vi "Encoders.vi"(0 "DigitalInputs":bool[](array[boolean])=[FALSE, FALSE, FALSE, FALSE, FALSE, FALSE, FALSE, FALSE, FALSE, FALSE, FALSE, FALSE, FALSE, FALSE, FALSE, FALSE, FALSE, FALSE, FALSE, FALSE, FALSE, FALSE, FALSE, FALSE, FALSE, FALSE, FALSE, FALSE, FALSE, FALSE, FALSE, FALSE], 1 "AnalogTriggers":T1[](array[typedef])=[{"InHysteresis"=FALSE, "OverLimit"=FALSE, "Rising"=FALSE, "Falling"=FALSE}, {"InHysteresis"=FALSE, "OverLimit"=FALSE, "Rising"=FALSE, "Falling"=FALSE}, {"InHysteresis"=FALSE, "OverLimit"=FALSE, "Rising"=FALSE, "Falling"=FALSE}, {"InHysteresis"=FALSE, "OverLimit"=FALSE, "Rising"=FALSE, "Falling"=FALSE}, {"InHysteresis"=FALSE, "OverLimit"=FALSE, "Rising"=FALSE, "Falling"=FALSE}, {"InHysteresis"=FALSE, "OverLimit"=FALSE, "Rising"=FALSE, "Falling"=FALSE}, {"InHysteresis"=FALSE, "OverLimit"=FALSE, "Rising"=FALSE, "Falling"=FALSE}, {"InHysteresis"=FALSE, "OverLimit"=FALSE, "Rising"=FALSE, "Falling"=FALSE}], 2 "Resets":T8, 3 "Configs":T9, 4 "TimerConfigs":T6) -> (5 "Outputs":T4, 6 "TimerOutputs":T2)   [LabVIEW 2019]
uses:
  Controls/Encoder_Configs.ctl
  Controls/Encoder_Config.ctl
  Helpers/Source.ctl
  Controls/Encoder_Resets.ctl
  Controls/Encoder_TimerConfigs.ctl
  Controls/TimerConfig.ctl
  Controls/Encoder_Outputs.ctl
  Controls/Encoder_Output.ctl
  Controls/Encoder_TimerOutputs.ctl
  Helpers/TimerOutput.ctl
  Helpers/AnalogTriggerOutput.ctl
  <vilib>/rvi/Emulation/niFpgaSctlEmulationGetInTimedLoop.vi
  <vilib>/rvi/Emulation/niFpgaProcessEmulError.vi
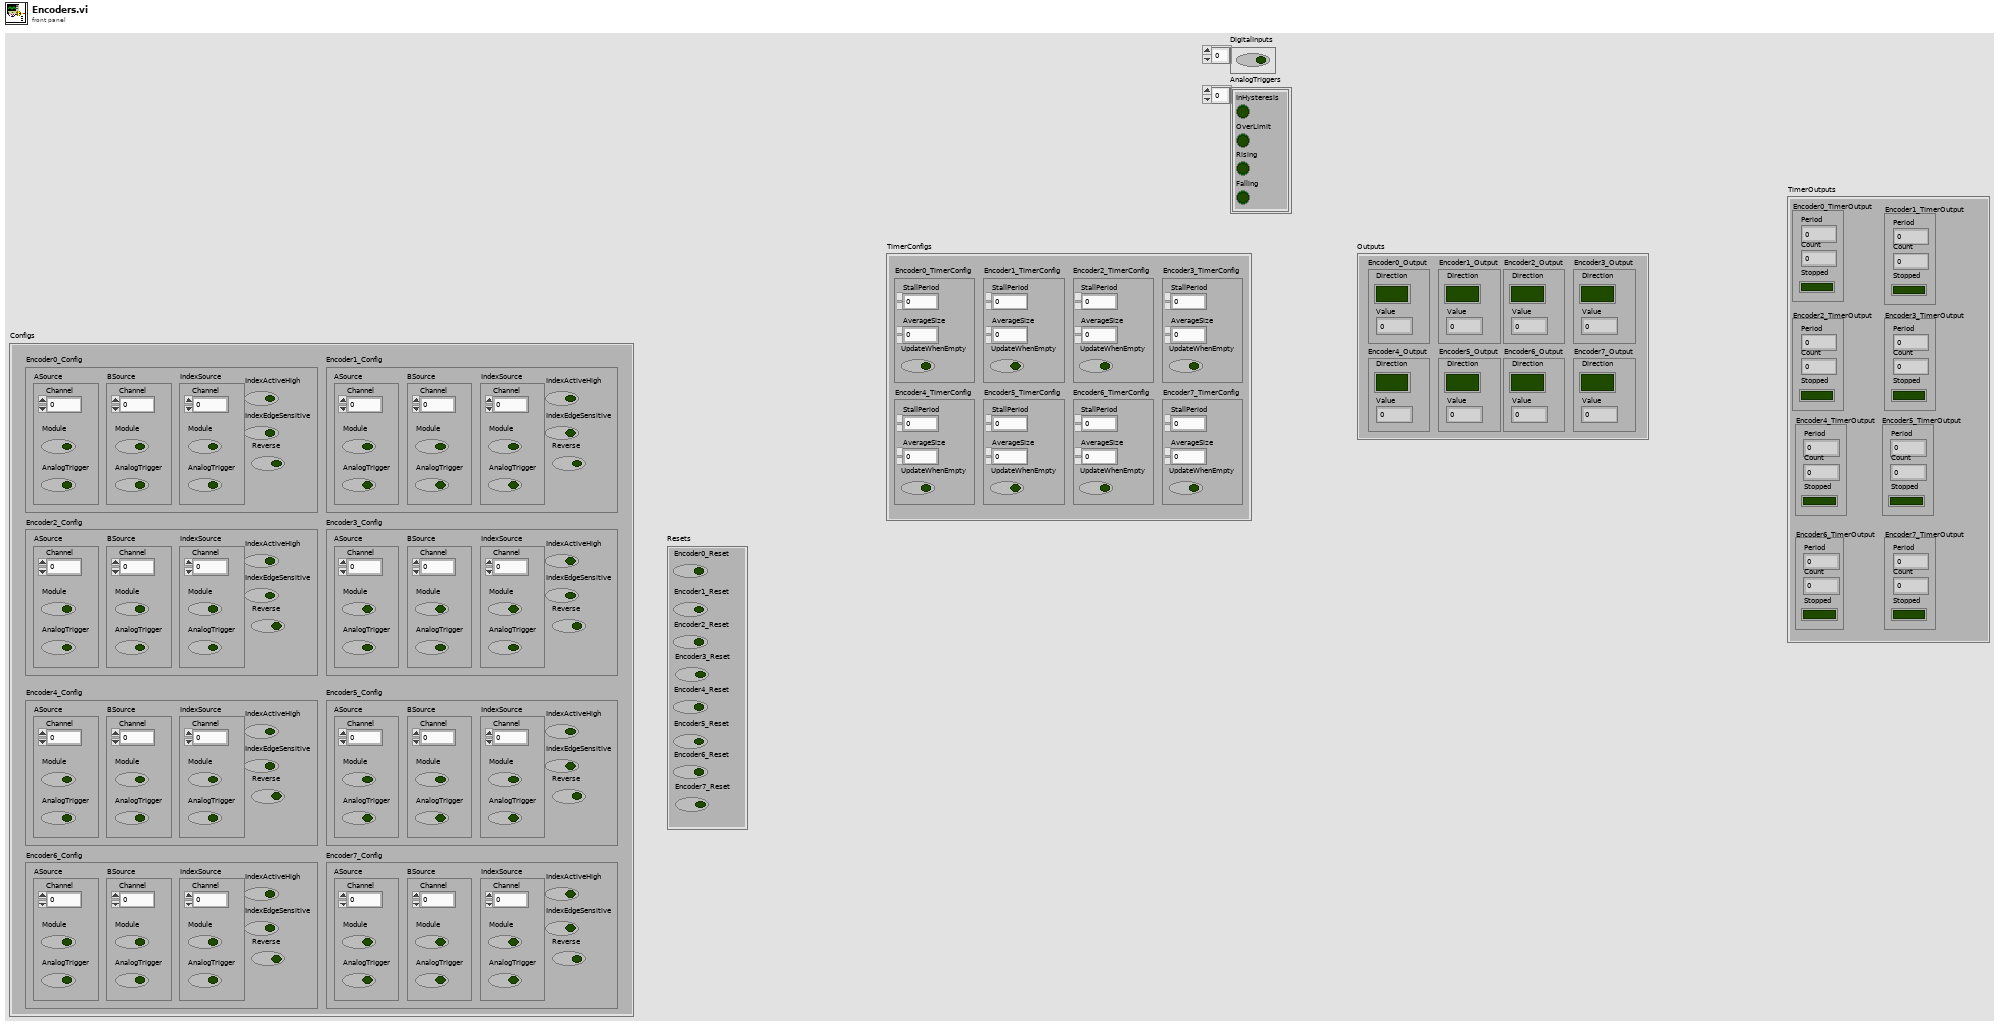
[diagram p1: front panel]
types:
  T1 = typedef "AnalogTriggerOutput.ctl" = cluster{"InHysteresis":bool, "OverLimit":bool, "Rising":bool, "Falling":bool}
  T2 = typedef "Encoder_TimerOutputs.ctl" = cluster{"Encoder0_TimerOutput":T3, "Encoder1_TimerOutput":T3, "Encoder2_TimerOutput":T3, "Encoder3_TimerOutput":T3, "Encoder4_TimerOutput":T3, "Encoder5_TimerOutput":T3, "Encoder6_TimerOutput":T3, "Encoder7_TimerOutput":T3}
  T3 = typedef "TimerOutput.ctl" = cluster{"Period":fxp<+,24,25>, "Count":i16, "Stopped":bool}
  T4 = typedef "Encoder_Outputs.ctl" = cluster{"Encoder0_Output":T5, "Encoder1_Output":T5, "Encoder2_Output":T5, "Encoder3_Output":T5, "Encoder4_Output":T5, "Encoder5_Output":T5, "Encoder6_Output":T5, "Encoder7_Output":T5}
  T5 = typedef "Encoder_Output.ctl" = cluster{"Direction":bool, "Value":fxp<+/-,31,31>}
  T6 = typedef "Encoder_TimerConfigs.ctl" = cluster{"Encoder0_TimerConfig":T7, "Encoder1_TimerConfig":T7, "Encoder2_TimerConfig":T7, "Encoder3_TimerConfig":T7, "Encoder4_TimerConfig":T7, "Encoder5_TimerConfig":T7, "Encoder6_TimerConfig":T7, "Encoder7_TimerConfig":T7}
  T7 = typedef "TimerConfig.ctl" = cluster{"StallPeriod":fxp<+,24,24>, "AverageSize":fxp<+,7,7>, "UpdateWhenEmpty":bool}
  T8 = typedef "Encoder_Resets.ctl" = cluster{"Encoder0_Reset":bool, "Encoder1_Reset":bool, "Encoder2_Reset":bool, "Encoder3_Reset":bool, "Encoder4_Reset":bool, "Encoder5_Reset":bool, "Encoder6_Reset":bool, "Encoder7_Reset":bool}
  T9 = typedef "Encoder_Configs.ctl" = cluster{"Encoder0_Config":T10, "Encoder1_Config":T10, "Encoder2_Config":T10, "Encoder3_Config":T10, "Encoder4_Config":T10, "Encoder5_Config":T10, "Encoder6_Config":T10, "Encoder7_Config":T10}
  T10 = typedef "Encoder_Config.ctl" = cluster{"ASource":T11, "BSource":T11, "IndexSource":T11, "IndexActiveHigh":bool, "IndexEdgeSensitive":bool, "Reverse":bool}
  T11 = typedef "Source.ctl" = cluster{"Channel":fxp<+,4,4>, "Module":bool, "AnalogTrigger":bool}
  T12 = typedef "CountingOutput.ctl" = cluster{"Direction":bool, "Value":fxp<+/-,31,31>}
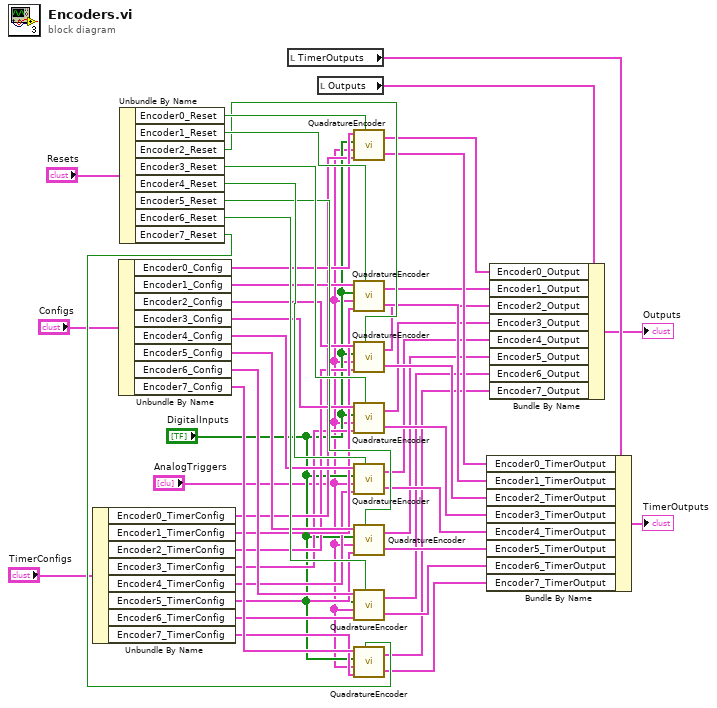
[diagram p0: block diagram]
diagram:
  n1 = Unbundle By Name("TimerConfigs") -> ("Encoder0_TimerConfig"=w30:T7, "Encoder1_TimerConfig"=w29:T7, "Encoder2_TimerConfig"=w28:T7, "Encoder3_TimerConfig"=w27:T7, "Encoder4_TimerConfig"=w26:T7, "Encoder5_TimerConfig"=w25:T7, "Encoder6_TimerConfig"=w24:T7, "Encoder7_TimerConfig"=w23:T7)
  n2 = Unbundle By Name("Configs") -> ("Encoder0_Config"=w39:T10, "Encoder1_Config"=w38:T10, "Encoder2_Config"=w37:T10, "Encoder3_Config"=w36:T10, "Encoder4_Config"=w35:T10, "Encoder5_Config"=w34:T10, "Encoder6_Config"=w33:T10, "Encoder7_Config"=w32:T10)
  n3 = Unbundle By Name("Resets") -> ("Encoder0_Reset"=w48:bool, "Encoder1_Reset"=w47:bool, "Encoder2_Reset"=w46:bool, "Encoder3_Reset"=w45:bool, "Encoder4_Reset"=w44:bool, "Encoder5_Reset"=w43:bool, "Encoder6_Reset"=w42:bool, "Encoder7_Reset"=w41:bool)
  n4 = local read "TimerOutputs"() -> (w20:T2)
  n5 = local read "Outputs"() -> (w9:T4)
  n6 = call "QuadratureEncoder.vi"("Reset"=w48, "TimerConfig"=w30, "AnalogTriggers"="AnalogTriggers", "DigitalInputs"="DigitalInputs", "Config"=w39) -> ("TimerOutput"=w18:T3, "Output"=w8:T12)  [unwired: 1 in]
  n7 = call "QuadratureEncoder.vi"("Reset"=w47, "TimerConfig"=w29, "AnalogTriggers"="AnalogTriggers", "DigitalInputs"="DigitalInputs", "Config"=w38) -> ("TimerOutput"=w17:T3, "Output"=w7:T12)  [unwired: 1 in]
  n8 = call "QuadratureEncoder.vi"("Reset"=w46, "TimerConfig"=w28, "AnalogTriggers"="AnalogTriggers", "DigitalInputs"="DigitalInputs", "Config"=w37) -> ("TimerOutput"=w16:T3, "Output"=w6:T12)  [unwired: 1 in]
  n9 = call "QuadratureEncoder.vi"("Reset"=w45, "TimerConfig"=w27, "AnalogTriggers"="AnalogTriggers", "DigitalInputs"="DigitalInputs", "Config"=w36) -> ("TimerOutput"=w15:T3, "Output"=w5:T12)  [unwired: 1 in]
  n10 = call "QuadratureEncoder.vi"("Reset"=w44, "TimerConfig"=w26, "AnalogTriggers"="AnalogTriggers", "DigitalInputs"="DigitalInputs", "Config"=w35) -> ("TimerOutput"=w14:T3, "Output"=w4:T12)  [unwired: 1 in]
  n11 = call "QuadratureEncoder.vi"("Reset"=w43, "TimerConfig"=w25, "AnalogTriggers"="AnalogTriggers", "DigitalInputs"="DigitalInputs", "Config"=w34) -> ("TimerOutput"=w13:T3, "Output"=w3:T12)  [unwired: 1 in]
  n12 = call "QuadratureEncoder.vi"("Reset"=w42, "TimerConfig"=w24, "AnalogTriggers"="AnalogTriggers", "DigitalInputs"="DigitalInputs", "Config"=w33) -> ("TimerOutput"=w12:T3, "Output"=w2:T12)  [unwired: 1 in]
  n13 = call "QuadratureEncoder.vi"("Reset"=w41, "TimerConfig"=w23, "AnalogTriggers"="AnalogTriggers", "DigitalInputs"="DigitalInputs", "Config"=w32) -> ("TimerOutput"=w11:T3, "Output"=w1:T12)  [unwired: 1 in]
  n14 = Bundle By Name(cluster=w20, "Encoder0_TimerOutput"=w18, "Encoder1_TimerOutput"=w17, "Encoder2_TimerOutput"=w16, "Encoder3_TimerOutput"=w15, "Encoder4_TimerOutput"=w14, "Encoder5_TimerOutput"=w13, "Encoder6_TimerOutput"=w12, "Encoder7_TimerOutput"=w11) -> (→"TimerOutputs":T2)
  n15 = Bundle By Name(cluster=w9, "Encoder0_Output"=w8, "Encoder1_Output"=w7, "Encoder2_Output"=w6, "Encoder3_Output"=w5, "Encoder4_Output"=w4, "Encoder5_Output"=w3, "Encoder6_Output"=w2, "Encoder7_Output"=w1) -> (→"Outputs":T4)
